vi "GetInitCamera.vi"(3 "LV_NumberSerial IN":u32, 4 "LV_SerialNumbers IN":u32[](array[numeric]), 5 "Selector":refnum<vi>) -> (0 "Hay Camaras?":bool, 1 "Camera Device OUT":T1, 2 "Camera Parameters OUT":T3 {"Pixel Format" items=["PIXEL_FORMAT_MONO8", "PIXEL_FORMAT_MONO16", "PIXEL_FORMAT_YUV422", "PIXEL_FORMAT_BAYER8_GRBG", "PIXEL_FORMAT_BAYER16_GRBG", "PIXEL_FORMAT_RGB24", "PIXEL_FORMAT_RGB48", "PIXEL_FORMAT_BAYER8_RGGB", "PIXEL_FORMAT_BAYER8_GBRG ", "PIXEL_FORMAT_BAYER8_BGGR ", "PIXEL_FORMAT_BAYER16_RGGB ", "PIXEL_FORMAT_BAYER16_GBRG", "PIXEL_FORMAT_BAYER16_BGGR", "PIXEL_FORMAT_RGB32"]})   [LabVIEW 2010]
uses:
  <vilib>/addons/PixeLINK/Low Level Functions/CAMERA_FEATURES.llb/TDPU-CameraFeatures-PixelFormat.ctl
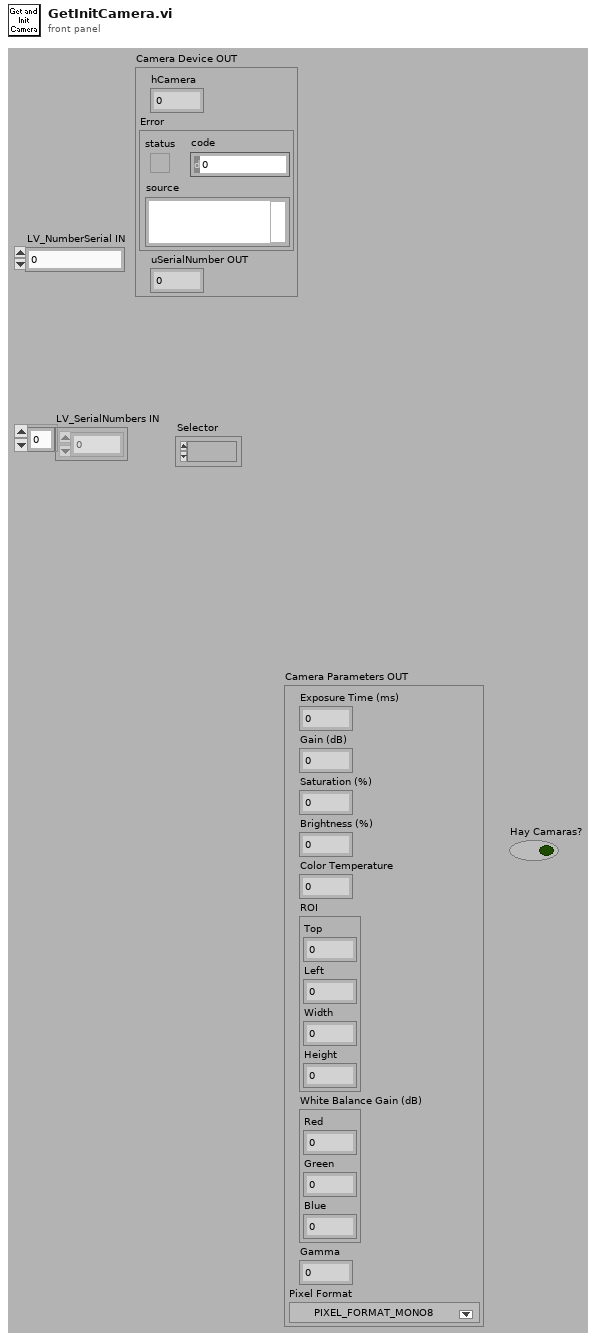
[diagram p1: front panel]
types:
  T1 = cluster{"hCamera":u32, "Error":errorcluster, "uSerialNumber OUT":u32}
  T2 = typedef "TDPU-CameraFeatures-PixelFormat.ctl" = u16
  T3 = cluster{"Exposure Time (ms)":dbl, "Gain (dB)":dbl, "Saturation (%)":dbl, "Brightness (%)":dbl, "Color Temperature":dbl, "ROI":cluster{"Top":i32, "Left":i32, "Width":i32, "Height":i32}, "White Balance Gain (dB)":cluster{"Red":dbl, "Green":dbl, "Blue":dbl}, "Gamma":dbl, "Pixel Format":T2}
  T4 = cluster{"hCamera":u32, "Error":errorcluster, "uSerialNumber":u32}
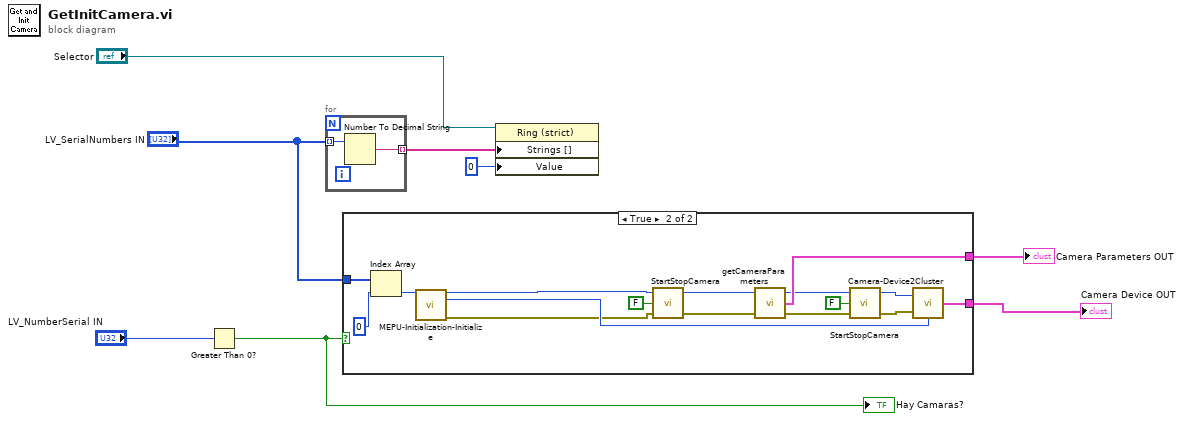
[diagram p0: block diagram]
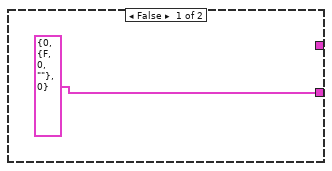
[diagram p2: hidden frame]
diagram:
  n1 = Greater Than 0?(x="LV_NumberSerial IN") -> (x > 0?=w7:bool)
  "Hay Camaras?" <- w7
  n2 = for {
    tunnel: [w10] -> w5 mode=indexing
    tunnel: "LV_SerialNumbers IN" -> [w9] mode=indexing
    n3 = Number To Decimal String(number=w9) -> (decimal integer string=w10:string)  [unwired: 1 in]
  }
  n4 = case shown="True" w7 {
    tunnel: "LV_SerialNumbers IN" -> [_ w27]
    tunnel: [T1 {"hCamera"=0, "Error"={"status"=FALSE, "code"=0, "source"=""}, "uSerialNumber OUT"=0} ("Camera Device OUT") w17] -> w1
    tunnel: [_ w25] -> w8
    frame False {
    }
    frame True {
      n5 = Index Array(array=w27, index=0) -> (element=w24:u32)
      n6 = call <vilib>:"MEPU-Initialization-Initialize.vi"("uSerialNumber IN"=w24) -> ("phCamera OUT"=w12:u32, "uSerialNumber OUT"=w18:u32, "Error OUT"=w13:errorcluster)  [unwired: 12 in]
      n7 = call "StartStopCamera.vi"("Error IN"=w13, "Camara ON?"=FALSE, "hCamera IN"=w12) -> ("Error OUT"=w16:errorcluster, "hCamera OUT"=w15:u32)  [unwired: 1 in]
      n8 = call "getCameraParameters.vi"("Error IN"=w16, "hCamera IN"=w15) -> ("Error OUT"=w20:errorcluster, "Camera Parameters"=w25:T3, "hCamera OUT"=w21:u32)  [unwired: 1 in]
      n9 = call "StartStopCamera.vi"("Error IN"=w20, "Camara ON?"=FALSE, "hCamera IN"=w21) -> ("Error OUT"=w22:errorcluster, "hCamera OUT"=w23:u32)  [unwired: 1 in]
      n10 = call "Camera-Device2Cluster.vi"("uSerialNumber IN"=w18, "Error IN"=w22, "hCamera IN"=w23) -> ("Camera Device OUT"=w17:T4)
    }
  }
  "Camera Parameters OUT" <- w8
  "Camera Device OUT" <- w1
  n11 = property on="Property Node" class="Ring (strict)"(reference="Selector", "Strings []"=w5, "Value"=0) -> ()  [unwired: 1 in, 2 out]
